vi "LNLS Control Send Command.vi"(7 "command body":string, 8 "error in (no error)":errorcluster, 9 "timeout ms (10000)":i32=10000, 10 "command ID":u8, 11 "connection ID":refnum<k5>) -> (0 "error out":errorcluster, 3 "connection ID out":refnum<k5>)   [LabVIEW 2011, in "LNLS Control VIs.lvlib"]
uses:
  LNLS Control VIs.lvlib
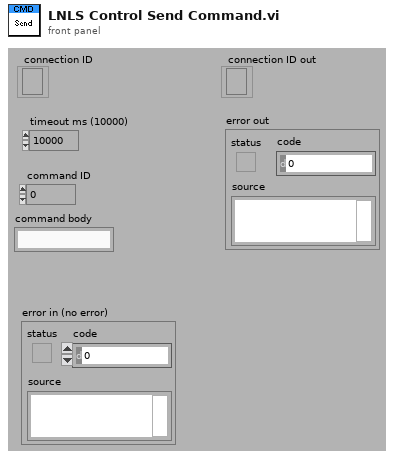
[diagram p1: front panel]
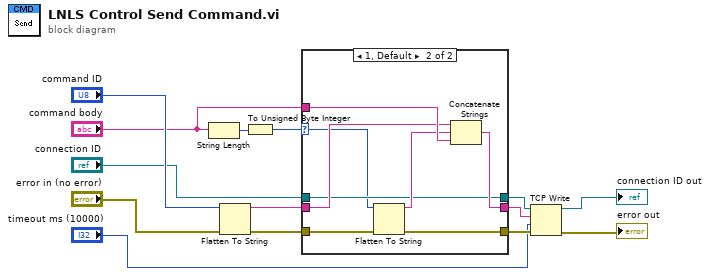
[diagram p0: block diagram]
diagram:
  n1 = String Length(string="command body") -> (length=w5:i32)
  n2 = Flatten To String(anything="command ID", error in (no error)="error in (no error)") -> (data string=w7:string, error out=w9:errorcluster)  [unwired: 2 in, 1 out]
  n3 = To Unsigned Byte Integer(number=w5) -> (unsigned 8bit integer=w4:u8)
  n4 = case shown="1, Default" w4 {
    selector: w4 -> [_ w18]
    tunnel: "command body" -> [_ w25]
    tunnel: w9 -> [w16 w24]
    tunnel: [w16 w23] -> w8
    tunnel: w7 -> [w15 w22]
    tunnel: [w15 w20] -> w6
    tunnel: [w17 w19] -> w3
    tunnel: "connection ID" -> [w17 w19]
    frame 0 {
    }
    frame 1, Default {
      n5 = Flatten To String(anything=w18, error in (no error)=w24) -> (data string=w21:string, error out=w23:errorcluster)  [unwired: 2 in, 1 out]
      n6 = Concatenate Strings(w22, w21, w25) -> (w20:string)
    }
  }
  n7 = TCP Write(connection ID=w3, data in=w6, error in (no error)=w8, 9:"timeout ms (10000)") -> (connection ID out=→"connection ID out":refnum<k5>, error out=→"error out":errorcluster)  [unwired: 1 out]
